vi "Periodic Tasks.vi"(8 "error in":errorcluster) -> ()   [LabVIEW 2014]
doc: "This VI runs in parallel to other tasks. It can contain as many user-defined periodic loops as you need. These can carry out PID or other sorts of timed response."
uses:
  <vilib>/Rock Robotics/SystemInterfaces/Utilities/FPGA_UtilitiesLED Source.ctl
  <vilib>/Rock Robotics/SystemInterfaces/Utilities/FPGA_UtilitiesLED State.ctl
  <vilib>/Rock Robotics/WPI/Compressor/WPI_CompressorGetSetRefNum.vi
  Robot Global Data.vi
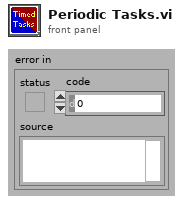
[diagram p1: front panel]
types:
  T1 = typedef "FPGA_UtilitiesLED State.ctl" = enum16{"Off", "On", "Toggle"}
  T2 = typedef "FPGA_UtilitiesLED Source.ctl" = enum16{"User LED", "FPGA LED"}
  T3 = cluster{"Trigger":bool, "Top 1":bool, "Side Trigger":bool, "Top 2":bool, "Top 3":bool, "Top 4":bool, "Bottom 1":bool, "Bottom 2":bool, "Bottom 3":bool, "Bottom 4":bool, "Bottom 5":bool, "Bottom 6":bool}
  T4 = typedef "WPI_CompressorDevRef.ctl" = cluster{"DevStatus":errorcluster, "DigitalInputDevRef":T5, "RelayDevRef":T8}
  T5 = typedef "WPI_DigitalInputDevRef.ctl" = cluster{"DevStatus":errorcluster, "DIO Channel":T6, "Digital Module":T7}
  T6 = typedef "FPGA_DIOChannel.ctl" = enum8{"DIO 1", "DIO 2", "DIO 3", "DIO 4", "DIO 5", "DIO 6", "DIO 7", "DIO 8", "DIO 9", "DIO 10", "DIO 11", "DIO 12", "DIO 13", "DIO 14", "Invalid"}
  T7 = typedef "FPGA_TypedefDigitalModule.ctl" = enum16{"Digital Module 1", "Digital Module 2"}
  T8 = typedef "WPI_RelayDevRef.ctl" = cluster{"DevStatus":errorcluster, "Relay Channel":T9, "Digital Module":T7, "Relay Direction":T10}
  T9 = typedef "FPGA_DIORelayChannel.ctl" = enum8{"Relay 1", "Relay 2", "Relay 3", "Relay 4", "Relay 5", "Relay 6", "Relay 7", "Relay 8", "Invalid"}
  T10 = typedef "WPI_RelayDirection.ctl" = enum16{"Both directions", "Forward only", "Reverse only"}
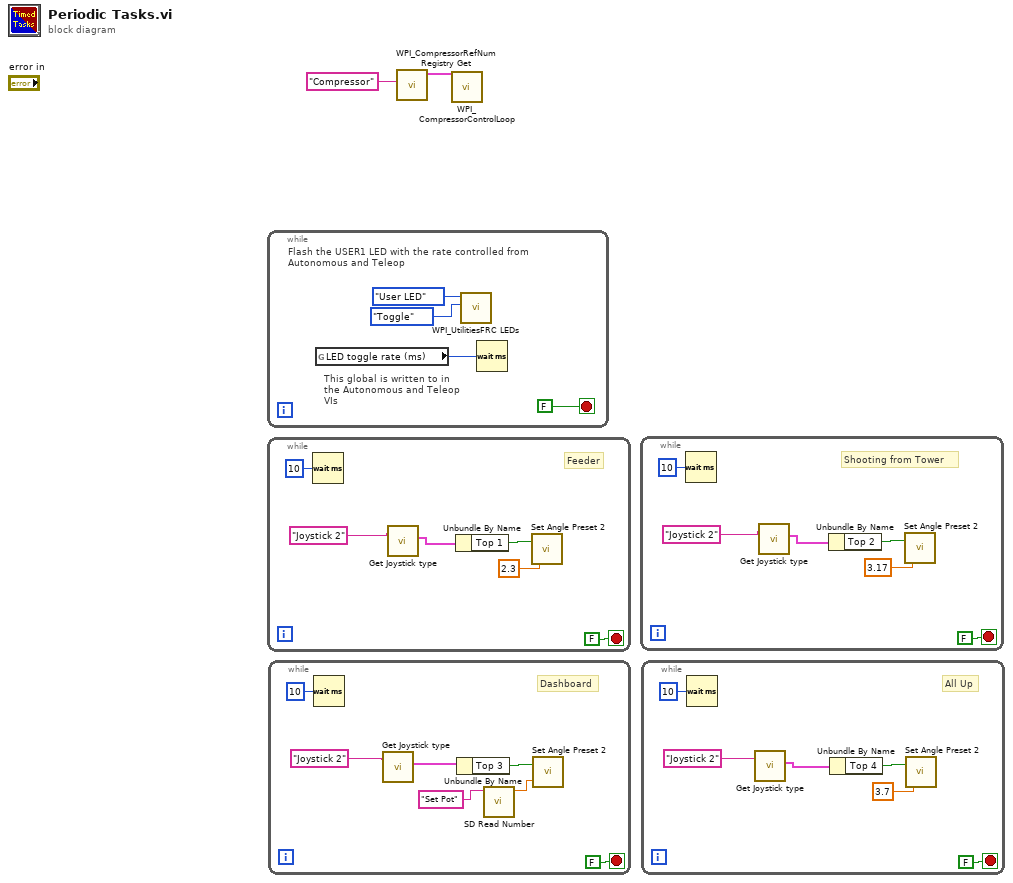
[diagram p0: block diagram]
diagram:
  n1 = while {
    stop <- FALSE stop-if-true
    # "This global is written to in the Autonomous and Teleop VIs"
    # "Flash the USER1 LED with the rate controlled from Autonomous and Teleop"
    n2 = global read "Robot Global Data.vi" "LED toggle rate (ms)"() -> (w3:u32)
    n3 = call <vilib>:"WPI_UtilitiesFRC LEDs.vi"("State"=FPGA_UtilitiesLED_State."Toggle", "LED Type"=FPGA_UtilitiesLED_Source."User LED") -> ()  [unwired: 1 in, 9 out]
    n4 = Wait (ms)(milliseconds to wait=w3) -> ()  [unwired: 1 out]
  }
  n5 = while {
    stop <- FALSE stop-if-true
    # "Feeder"
    n6 = Wait (ms)(milliseconds to wait=u32 10) -> ()  [unwired: 1 out]
    n7 = call "Get Joystick type.vi"("refnum name"="Joystick 2") -> ("Buttons"=w7:T3)  [unwired: 1 in, 3 out]
    n8 = Unbundle By Name(w7) -> ("Top 1"=w10:bool)
    n9 = call "Set Angle Preset 2.vi"("Set Angle"=2.3, "Enable"=w10) -> ()  [unwired: 1 in]
  }
  n10 = while {
    stop <- FALSE stop-if-true
    # "Dashboard"
    n11 = Wait (ms)(milliseconds to wait=u32 10) -> ()  [unwired: 1 out]
    n12 = call "Get Joystick type.vi"("refnum name"="Joystick 2") -> ("Buttons"=w13:T3)  [unwired: 1 in, 3 out]
    n13 = Unbundle By Name(w13) -> ("Top 3"=w17:bool)
    n14 = call <vilib>:"SD Read Number.vi"("Name"="Set Pot" ("refnum name")) -> ("Numeric"=w15:dbl)  [unwired: 8 in, 2 out]
    n15 = call "Set Angle Preset 2.vi"("Set Angle"=w15, "Enable"=w17) -> ()  [unwired: 1 in]
  }
  n16 = call <vilib>:"WPI_CompressorRefNum Registry Get.vi"("refnum name"="Compressor") -> ("CompressorDevRef"=w1:T4)  [unwired: 9 in, 1 out]
  n17 = call <vilib>:"WPI_CompressorControlLoop.vi"("CompressorDevRef"=w1) -> ()  [unwired: 11 in]
  n18 = while {
    stop <- FALSE stop-if-true
    # "Shooting from Tower"
    n19 = Wait (ms)(milliseconds to wait=u32 10) -> ()  [unwired: 1 out]
    n20 = call "Get Joystick type.vi"("refnum name"="Joystick 2") -> ("Buttons"=w20:T3)  [unwired: 1 in, 3 out]
    n21 = Unbundle By Name(w20) -> ("Top 2"=w23:bool)
    n22 = call "Set Angle Preset 2.vi"("Set Angle"=3.17, "Enable"=w23) -> ()  [unwired: 1 in]
  }
  n23 = while {
    stop <- FALSE stop-if-true
    # "All Up"
    n24 = Wait (ms)(milliseconds to wait=u32 10) -> ()  [unwired: 1 out]
    n25 = call "Get Joystick type.vi"("refnum name"="Joystick 2") -> ("Buttons"=w26:T3)  [unwired: 1 in, 3 out]
    n26 = Unbundle By Name(w26) -> ("Top 4"=w29:bool)
    n27 = call "Set Angle Preset 2.vi"("Set Angle"=3.7, "Enable"=w29) -> ()  [unwired: 1 in]
  }
